vi "read_params.vi"(8 "error in (no error)":errorcluster, 11 "NearestCentroid in":refnum<class "NearestCentroid.lvclass">) -> (0 "error out":errorcluster, 2 "params":T1={"metric"="euclidean", "shrink_threshold"={"shrink_threshold_type"="None", "shrink_threshold_float"=0.0}}, 3 "NearestCentroid out":refnum<class "NearestCentroid.lvclass">)   [LabVIEW 2020, in "NearestCentroid.lvclass"]
uses:
  NearestCentroid.lvclass
  Controls/nearest_centroid_params.ctl
  NearestCentroid.lvclass/NearestCentroid.ctl
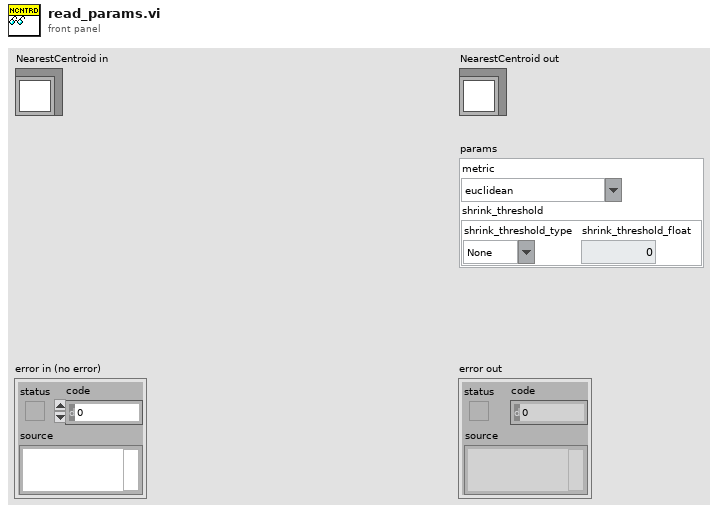
[diagram p1: front panel]
types:
  T1 = typedef "nearest_centroid_params.ctl" = cluster{"metric":string, "shrink_threshold":cluster{"shrink_threshold_type":string, "shrink_threshold_float":dbl}}
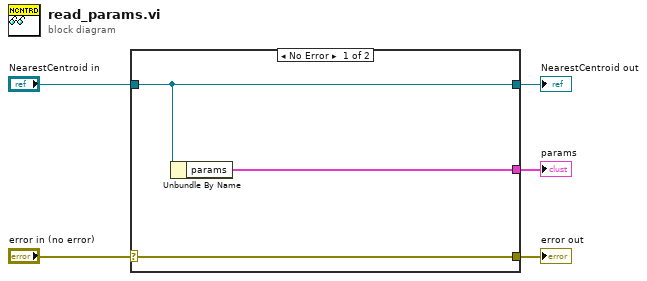
[diagram p0: block diagram]
diagram:
  n1 = case shown="No Error" "error in (no error)" {
    selector: "error in (no error)" -> [w8 w9]
    tunnel: [w8 w9] -> w4
    tunnel: [w7 w10] -> w2
    tunnel: "NearestCentroid in" -> [w7 w10]
    tunnel: [w6 _] -> w1
    frame No Error {
      n2 = Unbundle By Name(w7) -> ("params"=w6:T1)
    }
    frame Error {
    }
  }
  "error out" <- w4
  "NearestCentroid out" <- w2
  "params" <- w1
